vi "XNET.CAN.BusMonitor.Execute.vi"(8 "error in (no error)":errorcluster, 11 "gRPC Container in":refnum<class "XNET.CAN.BusMonitor.API.lvclass">) -> (0 "error out":errorcluster, 3 "gRPC Container out":refnum<class "XNET.CAN.BusMonitor.API.lvclass">)   [LabVIEW 2025, in "XNET.CAN.BusMonitor.API.lvlib" / "XNET.CAN.BusMonitor.API.lvclass"]
uses:
  XNET.CAN.BusMonitor.API.lvclass
  XNET.CAN.BusMonitor.API.lvclass/XNET.CAN.BusMonitor.API.ctl
  <vilib>/gRPC/LabVIEW gRPC Servicer/ServiceBase/ServiceBase.lvclass
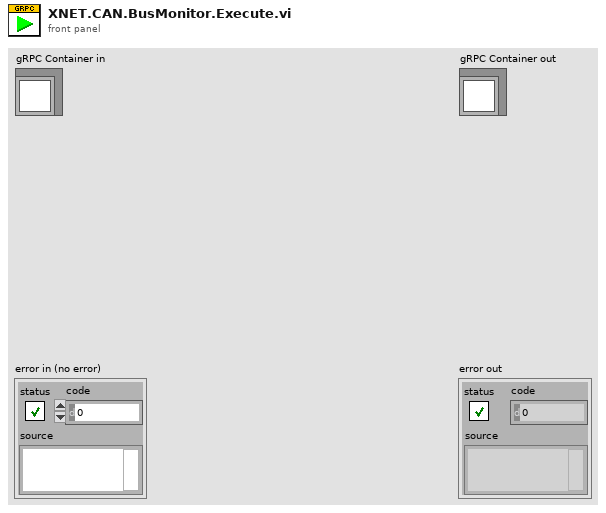
[diagram p1: front panel]
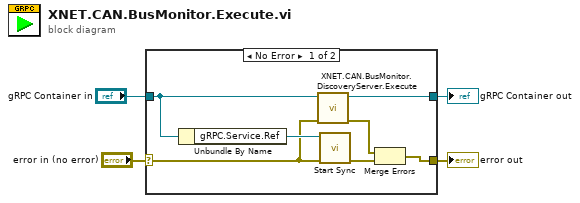
[diagram p0: block diagram]
diagram:
  n1 = case shown="No Error" "error in (no error)" {
    selector: "error in (no error)" -> [w8 w13]
    tunnel: [w9 w13] -> w3
    tunnel: [w6 w12] -> w1
    tunnel: "gRPC Container in" -> [w5 w12]
    frame No Error {
      n2 = Unbundle By Name(w5) -> ("gRPC.Service.Ref"=w10:refnum<class "ServiceBase.lvclass">)
      n3 = call "XNET.CAN.BusMonitor.DiscoveryServer.Execute.vi"("error in (no error)"=w8, "CAN.Streaming.API in"=w5) -> ("error out"=w7:errorcluster, "CAN.Streaming.API out"=w6:refnum<class "XNET.CAN.BusMonitor.API.lvclass">)  [unwired: 8 in]
      n4 = call-dynamic "Start Sync.vi"("error in"=w8, "gRPC service in"=w10) -> ("error out"=w11:errorcluster)  [unwired: 8 in, 1 out]
      n5 = Merge Errors(w7, w11) -> (w9:errorcluster)
    }
    frame Error {
    }
  }
  "error out" <- w3
  "gRPC Container out" <- w1
